vi "线段比例点.vi"(8 "Error In":errorcluster caption="错误输入", 9 "比例(CA/AB)":dbl=0.5, 10 "点B":T1, 11 "点A":T1) -> (0 "Error Out":errorcluster caption="错误输出", 3 "比例点":T1 caption="比例点C")   [LabVIEW 2012, in "几何工具.lvlib"]
uses:
  <vilib>/Utility/miscctls.llb/LVPointDoubleTypeDef.ctl
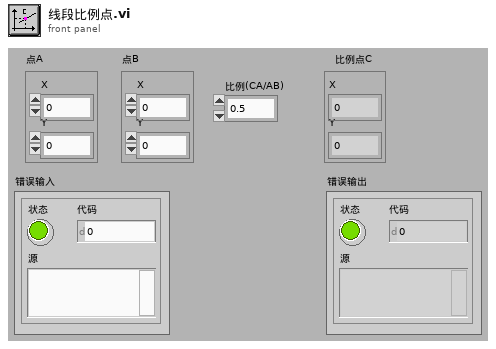
[diagram p1: front panel]
types:
  T1 = typedef "LVPointDoubleTypeDef.ctl" = cluster{"X":dbl, "Y":dbl}
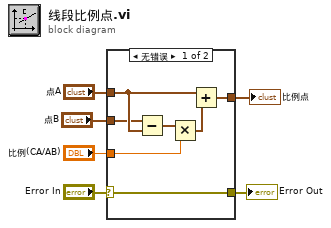
[diagram p0: block diagram]
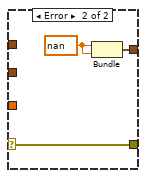
[diagram p2: hidden frame]
diagram:
  n1 = case shown="无错误" "Error In" {
    selector: "Error In" -> [w7 w16]
    tunnel: "点A" -> [w11 _]
    tunnel: "点B" -> [w10 _]
    tunnel: [w9 w14] -> w4
    tunnel: "比例(CA/AB)" -> [w8 _]
    tunnel: [w7 w16] -> w1
    frame No Error {
      n2 = Subtract(x=w10, y=w11) -> (x-y=w13:T1)
      n3 = Multiply(x=w13, y=w8) -> (x*y=w12:T1)
      n4 = Add(x=w11, y=w12) -> (x+y=w9:T1)
    }
    frame Error {
      w15 = nan
      n5 = Bundle(w15, w15) -> (w14:cluster{dbl, dbl})  [unwired: 1 in]
    }
  }
  "Error Out" <- w1
  "比例点" <- w4
